vi "Msg To Nested.vi"(8 "Alias":string, 9 "Priority Msg?":bool, 10 "Msg":refnum<class "Msg Strategy.lvclass">, 11 "Self Actor in":refnum<class "Self Actor.lvclass">) -> (0 "error out":errorcluster)   [LabVIEW 2021, in "jettl.lvlib" / "Self Actor.lvclass"]
uses:
  Self Actor.lvclass
  Msg Strategy/Msg Strategy.lvclass
  jettl.lvlib
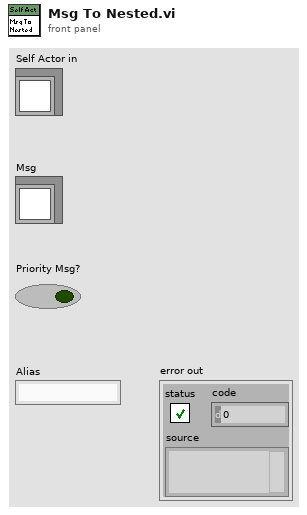
[diagram p1: front panel]
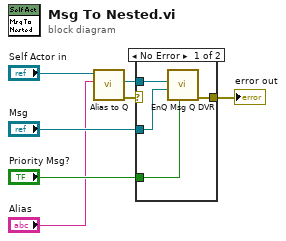
[diagram p0: block diagram]
diagram:
  n1 = call "Alias to Q.vi"("Msg Q DVR Alias"="Alias", "Self Actor in"="Self Actor in") -> ("error out"=w7:errorcluster, "Nested Msg Q DVR"=w6:refnum<data-value>)  [unwired: 8 in]
  n2 = case shown="No Error" w7 {
    selector: w7 -> [_ w12]
    tunnel: [w11 w12] -> w1
    tunnel: "Msg" -> [w10 _]
    tunnel: "Priority Msg?" -> [w9 _]
    tunnel: w6 -> [w8 _]
    frame No Error {
      n3 = call "EnQ Msg Q DVR.vi"("Priority Msg?"=w9, "Msg"=w10, "Msg Q DVR"=w8) -> ("error out"=w11:errorcluster)  [unwired: 8 in]
    }
    frame Error {
    }
  }
  "error out" <- w1
